vi "fire mech.vi"   [LabVIEW 2012]
uses:
  <vilib>/Rock Robotics/WPI/Solenoid/WPI_SolenoidValue.ctl
  <vilib>/Rock Robotics/WPI/Solenoid/WPI_SolenoidSetEnum.vi
types:
  T1 = typedef "WPI_JoystickDevRef.ctl" = cluster{"Device":T2}
  T2 = typedef "WPI_JoystickDeviceEnum.ctl" = enum16{"USB 1", "USB 2", "USB 3", "USB 4", "Kinect 1", "Kinect 2"}
  T3 = typedef "WPI_DigitalInputDevRef.ctl" = cluster{"DevStatus":errorcluster, "DIO Channel":T4, "Digital Module":T5}
  T4 = typedef "FPGA_DIOChannel.ctl" = enum8{"DIO 1", "DIO 2", "DIO 3", "DIO 4", "DIO 5", "DIO 6", "DIO 7", "DIO 8", "DIO 9", "DIO 10", "DIO 11", "DIO 12", "DIO 13", "DIO 14", "Invalid"}
  T5 = typedef "FPGA_TypedefDigitalModule.ctl" = enum16{"Digital Module 1", "Digital Module 2"}
  T6 = typedef "WPI_JoystickButtonState.ctl" = cluster{"Button 1":bool, "Button 2":bool, "Button 3":bool, "Button 4":bool, "Button 5":bool, "Button 6":bool, "Button 7":bool, "Button 8":bool, "Button 9":bool, "Button 10":bool, "Button 11":bool, "Button 12":bool}
  T7 = typedef "WPI_SolenoidDevRef.ctl" = cluster{"DevStatus":errorcluster, "Solenoid Module":T8, "Forward Solenoid Channel":T9, "Reverse Solenoid Channel":T9}
  T8 = typedef "FPGA_TypedefSolenoidModule.ctl" = enum16{"Solenoid Module 1", "Solenoid Module 2"}
  T9 = typedef "WPI_SolenoidChannel.ctl" = enum8{"Solenoid 1", "Solenoid 2", "Solenoid 3", "Solenoid 4", "Solenoid 5", "Solenoid 6", "Solenoid 7", "Solenoid 8", "Invalid"}
  T10 = typedef "WPI_SolenoidValue.ctl" = enum16{"Off", "On", "Forward", "Reverse"}
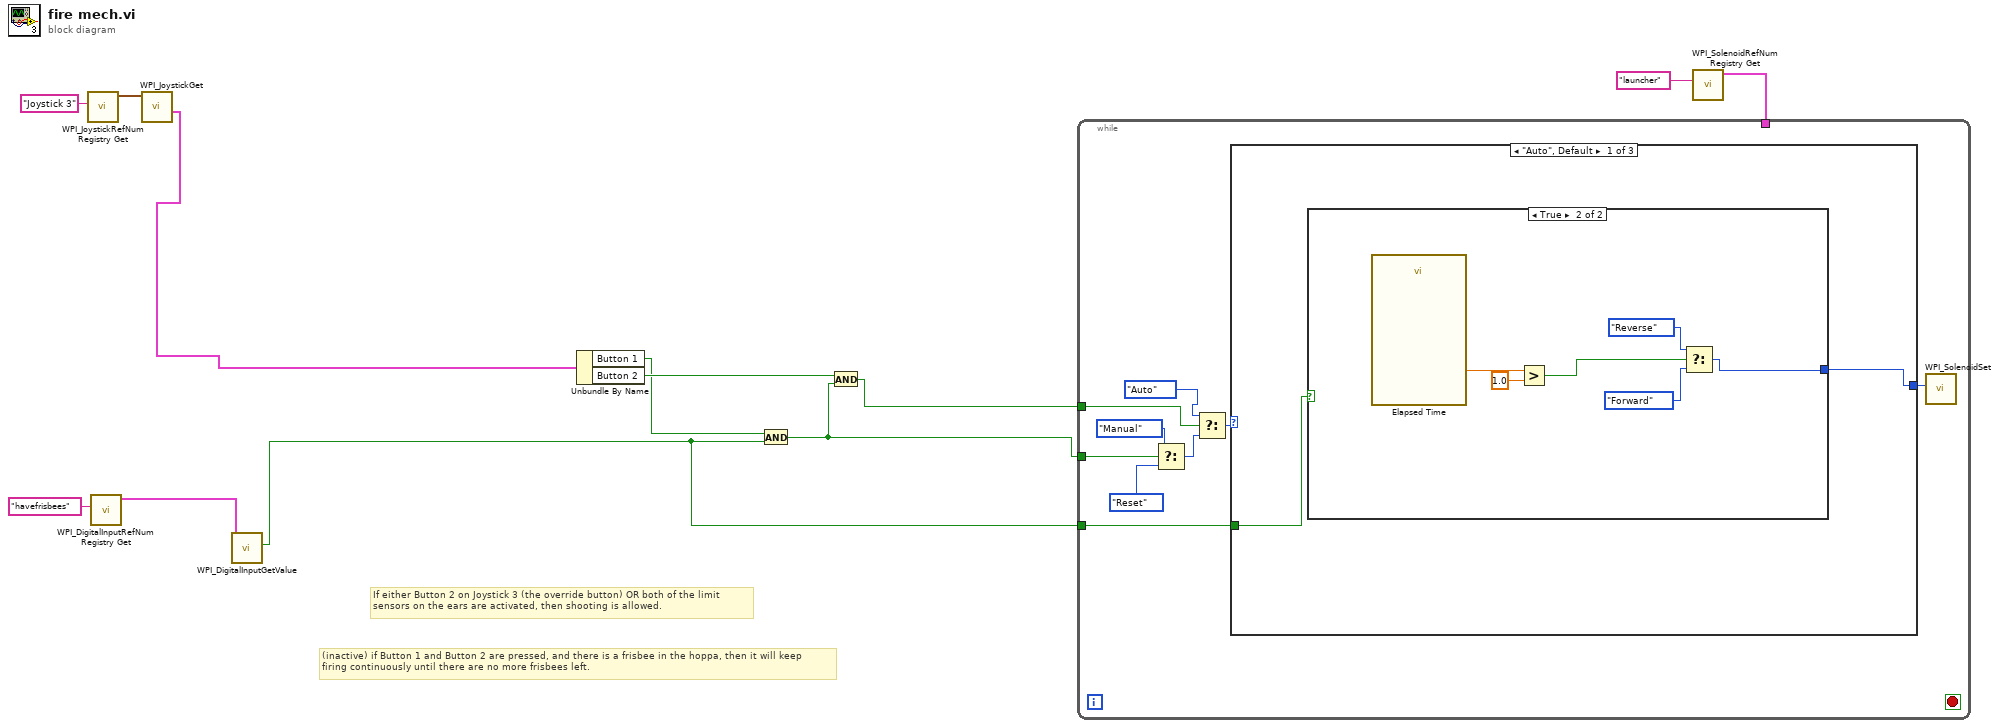
[diagram p0: block diagram]
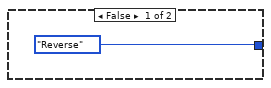
[diagram p2: hidden frame]
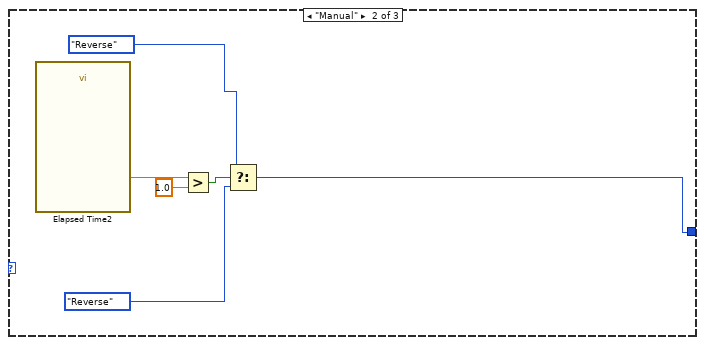
[diagram p3: hidden frame]
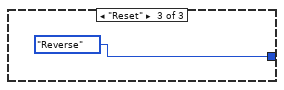
[diagram p4: hidden frame]
diagram:
  # "(inactive) if Button 1 and Button 2 are pressed, and there is a frisbee in the hoppa, then it will keep\nfiring continuously until there are no more frisbees left."
  # "If either Button 2 on Joystick 3 (the override button) OR both of the limit\nsensors on the ears are activated, then shooting is allowed."
  n1 = call <vilib>:"WPI_JoystickRefNum Registry Get.vi"("refnum name"="Joystick 3") -> ("JoystickDevRef"=w2:T1)  [unwired: 1 in, 9 out]
  n2 = call <vilib>:"WPI_DigitalInputRefNum Registry Get.vi"("refnum name"="havefrisbees") -> ("DigitalInputDevRef"=w6:T3)  [unwired: 9 in, 1 out]
  n3 = call <vilib>:"WPI_JoystickGet.vi"("JoystickDevRef"=w2) -> ("Buttons"=w3:T6)  [unwired: 1 in, 5 out]
  n4 = call <vilib>:"WPI_DigitalInputGetValue.vi"("DigitalInputDevRef"=w6) -> ("Value"=w12:bool)  [unwired: 8 in, 2 out]
  n5 = Unbundle By Name(w3) -> ("Button 1"=w4:bool, "Button 2"=w10:bool)
  n6 = And(x=w4, y=w12) -> (x .and. y?=w9:bool)
  n7 = And(x=w10, y=w9) -> (x .and. y?=w11:bool)
  n8 = call <vilib>:"WPI_SolenoidRefNum Registry Get.vi"("refnum name"="launcher") -> ("SolenoidDevRef"=w7:T7)  [unwired: 9 in, 1 out]
  n9 = while {
    tunnel: w7 -> [_]
    tunnel: w9 -> [w16]
    tunnel: w11 -> [w15]
    tunnel: w12 -> [w13]
    stop <- _ stop-if-true
    n10 = Select(t=enum16{"Auto", "Reset", "Manual"}."Manual", s=w16, f=enum16{"Auto", "Reset", "Manual"}."Reset") -> (s? t:f=w21:enum16{"Auto", "Reset", "Manual"})
    n11 = Select(t=enum16{"Auto", "Reset", "Manual"}."Auto", s=w15, f=w21) -> (s? t:f=w17:enum16{"Auto", "Reset", "Manual"})
    n12 = case shown="\"Auto\", Default" w17 {
      tunnel: [w23 w34 WPI_SolenoidValue."Reverse" ("Value")] -> w14
      tunnel: w13 -> [w22 _ _]
      frame "Auto", Default {
        n13 = case shown="True" w22 {
          tunnel: [WPI_SolenoidValue."Reverse" ("Value") w28] -> w23
          frame False {
          }
          frame True {
            n14 = call "Elapsed Time"() -> ("Elapsed Time (s)"=w27:dbl)  [unwired: 12 in, 7 out]
            n15 = Greater?(x=w27, y=1.0) -> (0:w25:bool)
            n16 = Select(t=WPI_SolenoidValue."Reverse" ("Value"), s=w25, f=WPI_SolenoidValue."Forward" ("Value")) -> (s? t:f=w28:T10)
          }
        }
      }
      frame "Manual" {
        n17 = call "Elapsed Time2"() -> ("Elapsed Time (s)"=w33:dbl)  [unwired: 12 in, 7 out]
        n18 = Greater?(x=w33, y=1.0) -> (0:w31:bool)
        n19 = Select(t=WPI_SolenoidValue."Reverse" ("Value"), s=w31, f=WPI_SolenoidValue."Reverse" ("Value")) -> (s? t:f=w34:T10)
      }
      frame "Reset" {
      }
    }
    n20 = call-poly <vilib>:"WPI_SolenoidSet.vi"("Value"=w14) -> ()  [unwired: 9 in, 2 out]
  }
